vi "initialize.vi"(8 "error in (no error)":errorcluster, 11 "Pfeiffer MultiGauge TPG256 in":refnum<class "Pfeiffer MultiGauge TPG256.lvclass">) -> (0 "error out":errorcluster, 1 "Programm version":string, 2 "initialized?":bool, 3 "Pfeiffer MultiGauge TPG256 out":refnum<class "Pfeiffer MultiGauge TPG256.lvclass">)   [LabVIEW 2018, in "Pfeiffer MultiGauge TPG256.lvclass"]
doc: "initializes an instrument; this method is going to be replaced by the same method of the child objects"
uses:
  Pfeiffer MultiGauge TPG256.lvclass
  instrument.lvclass
  Drivers/Pfeiffer_MaxiGauge/Maxi Gauge.lvlib
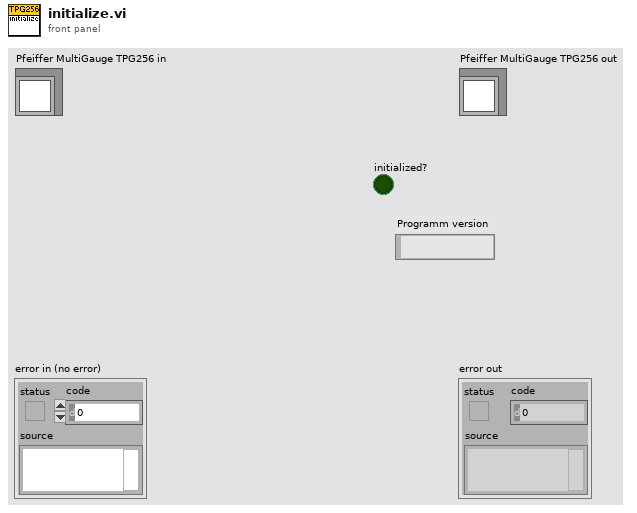
[diagram p1: front panel]
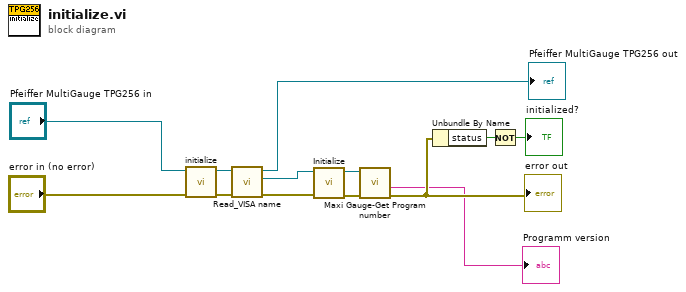
[diagram p0: block diagram]
diagram:
  n1 = call-parent "initialize.vi"("error in (no error)"="error in (no error)", "instrument in"="Pfeiffer MultiGauge TPG256 in") -> ("error out"=w10:errorcluster, "instrument out"=w11:refnum<class "Pfeiffer MultiGauge TPG256.lvclass">)  [unwired: 6 in, 2 out]
  n2 = call-dynamic "Read_VISA name.vi"("error in (no error)"=w10, "instrument in"=w11) -> ("error out"=w8:errorcluster, "VISA resource name"=w7:refnum<visa-resource-name>, "instrument out"=→"Pfeiffer MultiGauge TPG256 out":refnum<class "Pfeiffer MultiGauge TPG256.lvclass">)  [unwired: 7 in]
  n3 = call "Initialize.vi"("error in (no error)"=w8, "input refnum"=w7) -> ("error out"=w3:errorcluster, "VISA resource out"=w4:refnum<visa-resource-name>)  [unwired: 8 in]
  n4 = call "Maxi Gauge-Get Program number.vi"("Fehler (Eingang)"=w3, "VISA-Ressource in"=w4) -> ("Fehler (Ausgang)"=w2:errorcluster, "Programm version"=→"Programm version":string)  [unwired: 7 in, 1 out]
  "error out" <- w2
  n5 = Unbundle By Name(w2) -> ("status"=w6:bool)
  n6 = Not(x=w6) -> (.not. x?=→"initialized?":bool)
